vi "Close View FP.vi"(0 "GUI Container Actor in":refnum<class "GUI Container Actor.lvclass">, 5 "View":string, 7 "View Hierarchy Level":i32, 11 "error in (no error)":errorcluster) -> (4 "GUI Container Actor out":refnum<class "GUI Container Actor.lvclass">, 15 "error out":errorcluster)   [LabVIEW 2017, in "GUI Views.lvlib" / "GUI Container Actor.lvclass"]
doc: "Closes the Front Panel of a specified Actor Core VI of the the specified View class hierarchy. The Front Panel is specified by: \n\n<b> View </b> String theat contains the name of the View\n\n<b> View Hierarchy Level</b> the level on the subclassing hierarchy of the GUI View actor, it is used to choose the Actor Core Front Panel among all the exisiting sublcasses of the GUI VIew Actor present in the View specified above"
uses:
  GUI Container Actor.lvclass
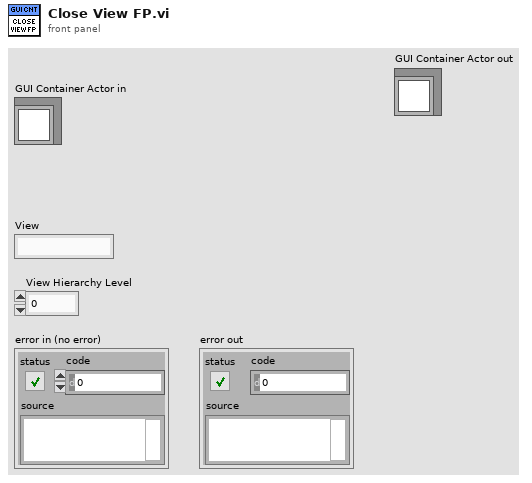
[diagram p1: front panel]
types:
  T1 = typedef "GUI Views.lvlib/GUI Container Actor.lvclass/View Status.ctl" = cluster{"View Details":T2, "Front Panel Statuses":T3[]}
  T2 = typedef "GUI Views.lvlib/GUI Container Actor.lvclass/View Details.ctl" = cluster{"Enqueuer":refnum<class "Message Enqueuer.lvclass">, "VI References":refnum<vi>[], "FP References":refnum<vi>[]}
  T3 = typedef "GUI Views.lvlib/GUI Container Actor.lvclass/FP Status.ctl" = cluster{"FP Open":bool, "Inserted in Subpanel":bool, "Subpanel":string}
  T4 = typedef "GUI Views.lvlib/GUI Container Actor.lvclass/VI References.ctl" = cluster{"FP Ref":refnum<vi>, "VI Ref":refnum<vi>}
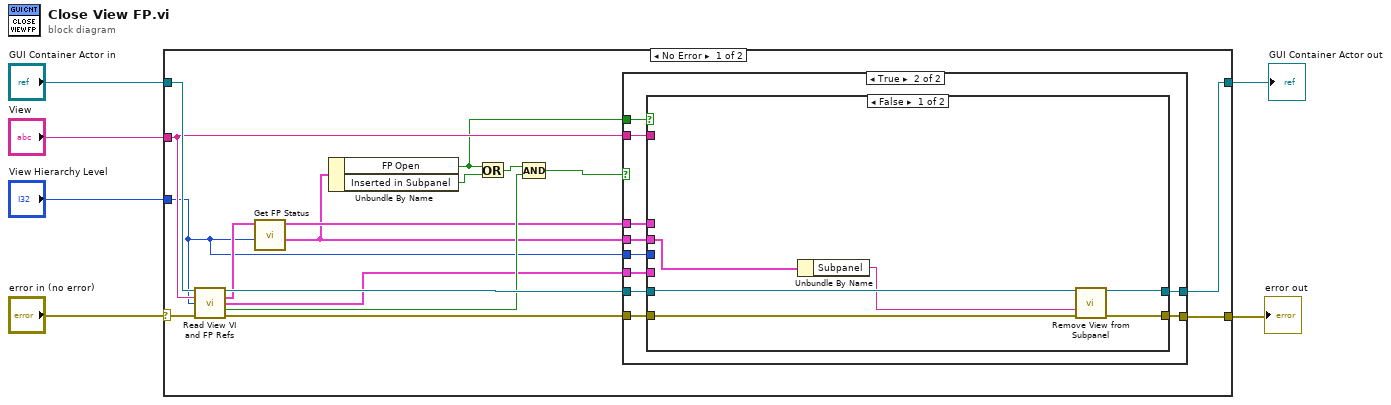
[diagram p0: block diagram]
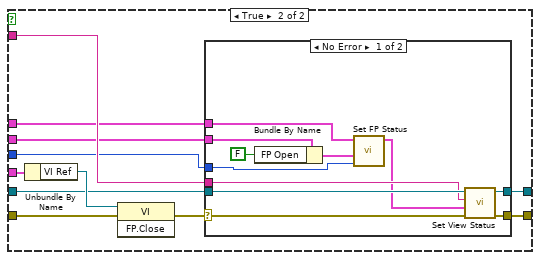
[diagram p3: hidden frame]
diagram:
  n1 = case shown="No Error" "error in (no error)" {
    selector: "error in (no error)" -> [w22 w66]
    tunnel: [w23 w66] -> w6
    tunnel: "GUI Container Actor in" -> [w20 w67]
    tunnel: "View Hierarchy Level" -> [w10 _]
    tunnel: "View" -> [w15 _]
    tunnel: [w14 w67] -> w1
    frame No Error {
      n2 = call "Read View VI and FP Refs.vi"("GUI Container Actor in"=w20, "View"=w15, "View Hierarchy Level"=w10, "error in (no error)"=w22) -> ("GUI Container Actor out"=w19:refnum<class "GUI Container Actor.lvclass">, "View Status"=w13:T1, "VI References"=w16:T4, "View Found"=w18:bool, "error out"=w21:errorcluster)  [unwired: 7 in]
      n3 = call "Get FP Status.vi"("View Hierarchy Level"=w10, "View Status in"=w13) -> ("FP Status"=w11:T3, "View Status out"=w12:T1)  [unwired: 8 in]
      n4 = Unbundle By Name(w11) -> ("FP Open"=w7:bool, "Inserted in Subpanel"=w8:bool)
      n5 = Or(x=w7, y=w8) -> (x .or. y?=w9:bool)
      n6 = Compound Arithmetic op=AND(w9, w18) -> (w17:bool)
      n7 = case shown="True" w17 {
        tunnel: [w25 w33] -> w23
        tunnel: w21 -> [w25 w35]
        tunnel: w19 -> [w24 w32]
        tunnel: w16 -> [_ w34]
        tunnel: w15 -> [_ w31]
        tunnel: [w24 w30] -> w14
        tunnel: w12 -> [_ w27]
        tunnel: w11 -> [_ w29]
        tunnel: w10 -> [_ w28]
        tunnel: w7 -> [_ w26]
        frame False {
        }
        frame True {
          n8 = case shown="False" w26 {
            tunnel: w35 -> [w41 w52]
            tunnel: w34 -> [_ w51]
            tunnel: [w40 w49] -> w33
            tunnel: w32 -> [w38 w48]
            tunnel: w31 -> [_ w46]
            tunnel: [w39 w45] -> w30
            tunnel: w29 -> [w37 w44]
            tunnel: w28 -> [_ w43]
            tunnel: w27 -> [_ w42]
            frame False {
              n9 = Unbundle By Name(w37) -> ("Subpanel"=w36:string)
              n10 = call "Remove View from Subpanel.vi"("GUI Container Actor in"=w38, "Subpanel"=w36, "error in (no error)"=w41) -> ("GUI Container Actor out"=w39:refnum<class "GUI Container Actor.lvclass">, "error out"=w40:errorcluster)  [unwired: 11 in]
            }
            frame True {
              n11 = Unbundle By Name(w51) -> ("VI Ref"=w50:refnum<vi>)
              n12 = invoke class="VI" method="FP.Close"(reference=w50, error in=w52) -> (error out=w47:errorcluster)  [unwired: 1 in, 2 out]
              n13 = case shown="No Error" w47 {
                selector: w47 -> [w61 w65]
                tunnel: [w63 w65] -> w49
                tunnel: w48 -> [w62 w64]
                tunnel: w46 -> [w59 _]
                tunnel: [w58 w64] -> w45
                tunnel: w44 -> [w57 _]
                tunnel: w43 -> [w56 _]
                tunnel: w42 -> [w55 _]
                frame No Error {
                  n14 = Bundle By Name(cluster=w57, "FP Open"=FALSE) -> (w53:T3)
                  n15 = call "Set FP Status.vi"("View Hierarchy Level"=w56, "FP Status"=w53, "View Status in"=w55) -> ("View Status out"=w54:T1)  [unwired: 8 in]
                  n16 = call "Set View Status.vi"("error in (no error)"=w61, "View Status"=w54, "View"=w59, "GUI Container Actor in"=w62) -> ("error out"=w63:errorcluster, "GUI Container Actor out"=w58:refnum<class "GUI Container Actor.lvclass">)  [unwired: 5 in, 1 out]
                }
                frame Error {
                }
              }
            }
          }
        }
      }
    }
    frame Error {
    }
  }
  "error out" <- w6
  "GUI Container Actor out" <- w1
